vi "Configure Numeric.vi"(5 "element":u16(ring) items=["1", "2", "3", "4", "5", "6", "7", "SIGMA", "SIGMB", "SIGMC"], 7 "function":u16(ring) items=["Urms", "Irms", "P", "S", "Q"], 8 "error in（no error）":errorcluster, 10 "item":u32=1 min=1 max=255 step=1, 11 "VISA resource name":refnum<visa-resource-name>) -> (0 "error out":errorcluster, 3 "VISA resource out":refnum<visa-resource-name>)   [LabVIEW 2018, in "Suita SPAW7000.lvlib"]
uses:
  <instrlib>/Suita SPAW7000/Suita SPAW7000.lvlib
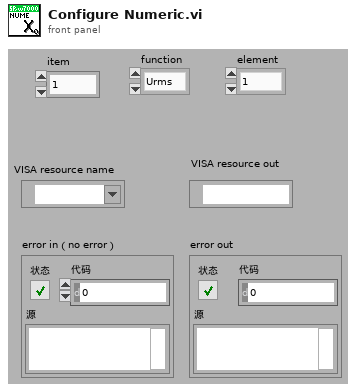
[diagram p1: front panel]
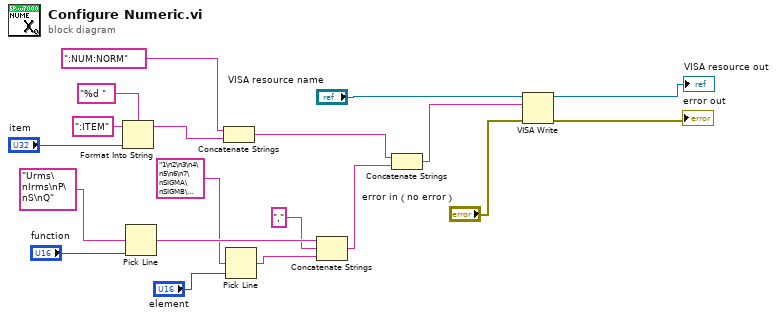
[diagram p0: block diagram]
diagram:
  n1 = Format Into String(format string="%d " ("格式字符串"), initial string=":ITEM" ("初始字符串"), "item") -> (resulting string=w15:string)  [unwired: 1 in, 1 out]
  n2 = Pick Line(multi-line string="Urms\nIrms\nP\nS\nQ", line index="function") -> (output string=w11:string)  [unwired: 1 in]
  n3 = Concatenate Strings(":NUM:NORM", w15) -> (w8:string)
  n4 = Pick Line(multi-line string="1\n2\n3\n4\n5\n6\n7\nSIGMA\nSIGMB\nSIGMC", line index="element") -> (output string=w4:string)  [unwired: 1 in]
  n5 = Concatenate Strings(w11, "," ("字符串"), w4) -> (w7:string)
  n6 = Concatenate Strings(w8, w7) -> (w6:string)
  n7 = VISA Write(VISA resource name="VISA resource name", write buffer=w6, error in (no error)="error in（no error）") -> (VISA resource name out=→"VISA resource out":refnum<visa-resource-name>, error out=→"error out":errorcluster)  [unwired: 1 out]
